vi "ConnectToScopeAndGenerator.vi"(11 "Input Number":dbl) -> (0 "GEN error out":errorcluster, 1 "GEN resource output":refnum<visa-resource-name>, 2 "OSC error out":errorcluster, 3 "OSC Reference":refnum<visa-resource-name>)   [LabVIEW 2021]
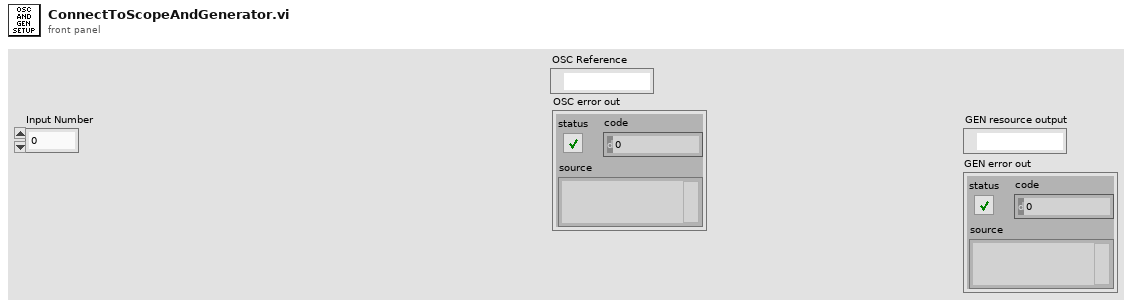
[diagram p1: front panel]
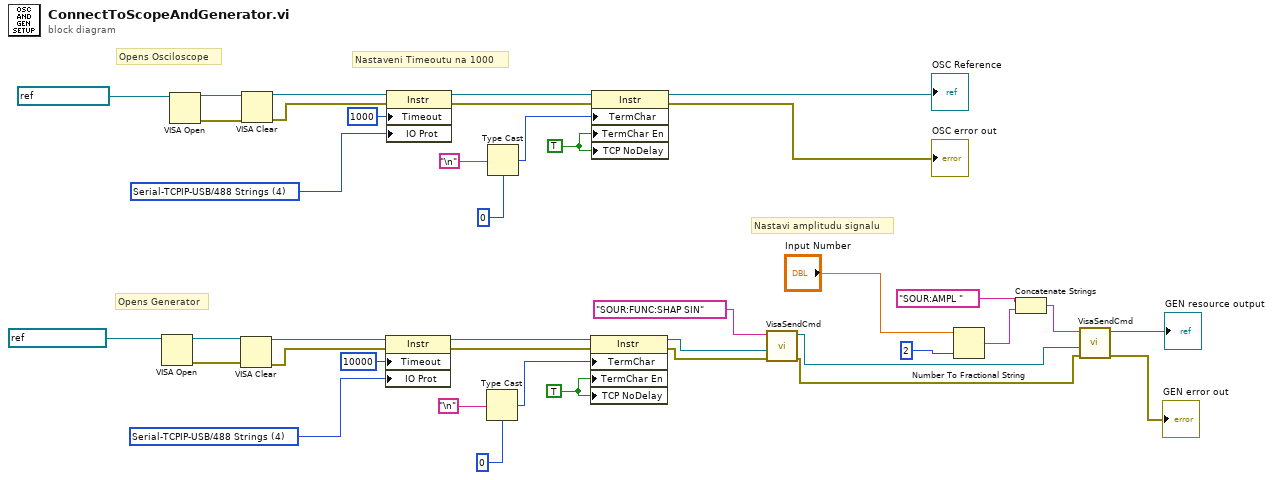
[diagram p0: block diagram]
diagram:
  w16 = TRUE
  w20 = u16 4 items=["Normal"=1, "VXI/FDC"=2, "GPIB/HS488"=3, "Serial-TCPIP-USB/488 Strings"=4, "USBTMC/Vendor-Specific"=5] ("Message Based Settings:IO Protocol")
  w28 = TRUE
  w32 = u16 4 items=["Normal"=1, "VXI/FDC"=2, "GPIB/HS488"=3, "Serial-TCPIP-USB/488 Strings"=4, "USBTMC/Vendor-Specific"=5] ("Message Based Settings:IO Protocol")
  # "Nastavi amplitudu signalu"
  # "Opens Generator"
  # "Nastaveni Timeoutu na 1000"
  # "Opens Osciloscope"
  n1 = VISA Open(VISA resource name=refnum<visa-resource-name> "FG_Simulator") -> (VISA resource name=w14:refnum<visa-resource-name>, error out=w13:errorcluster)  [unwired: 4 in]
  n2 = VISA Open(VISA resource name=refnum<visa-resource-name> "Osciloscope") -> (VISA resource name=w39:refnum<visa-resource-name>, error out=w38:errorcluster)  [unwired: 4 in]
  n3 = VISA Clear(VISA resource name=w14, error in (no error)=w13) -> (VISA resource name out=w25:refnum<visa-resource-name>, error out=w24:errorcluster)
  n4 = VISA Clear(VISA resource name=w39, error in (no error)=w38) -> (VISA resource name out=w37:refnum<visa-resource-name>, error out=w36:errorcluster)
  n5 = property class="Instr"(reference=w25, error in=w24, "Timeout"=u32 10000 ("General Settings:Timeout Value"), "IO Prot"=w20) -> (reference out=w23:refnum<visa-resource-name>, error out=w22:errorcluster)
  n6 = property class="Instr"(reference=w37, error in=w36, "Timeout"=u32 1000 ("General Settings:Timeout Value"), "IO Prot"=w32) -> (reference out=w35:refnum<visa-resource-name>, error out=w34:errorcluster)
  n7 = Type Cast(type=0, x="\n") -> (*(type *) &x=w17:i32)
  n8 = Type Cast(type=0, x="\n") -> (*(type *) &x=w29:i32)
  n9 = property class="Instr"(reference=w23, error in=w22, "TermChar"=w17, "TermChar En"=w16, "TCP NoDelay"=w16) -> (reference out=w11:refnum<visa-resource-name>, error out=w10:errorcluster)
  n10 = property class="Instr"(reference=w35, error in=w34, "TermChar"=w29, "TermChar En"=w28, "TCP NoDelay"=w28) -> (reference out=→"OSC Reference":refnum<visa-resource-name>, error out=→"OSC error out":errorcluster)
  n11 = call "VisaSendCmd.vi"("error in (no error)"=w10, "VISA resource name"=w11, "Msg to send"="SOUR:FUNC:SHAP SIN") -> ("error out"=w4:errorcluster, "VISA resource output"=w5:refnum<visa-resource-name>)  [unwired: 7 in]
  n12 = Number To Fractional String(number="Input Number", precision (6)=i16 2) -> (F-format string=w8:string)  [unwired: 2 in]
  n13 = Concatenate Strings("SOUR:AMPL ", w8) -> (w6:string)
  n14 = call "VisaSendCmd.vi"("error in (no error)"=w4, "VISA resource name"=w5, "Msg to send"=w6) -> ("error out"=→"GEN error out":errorcluster, "VISA resource output"=→"GEN resource output":refnum<visa-resource-name>)  [unwired: 7 in]
